vi "SDG60DeleteAllWaveforms.vi"(2 "error in (no error)":errorcluster, 4 "VISA resource name":refnum<visa-resource-name>="USB0::0xF4EC::0x1101::SDG6XEBC5R0119::INSTR") -> (0 "error out":errorcluster, 1 "VISA resource name out":refnum<visa-resource-name>, 3 "Time Estimation (s)":i32=7 format="%.15f")   [LabVIEW 2018]
doc: "Establishes communication with the instrument and optionally performs an instrument identification query and/or an instrument reset. It also places the instrument in a default state needed for other instrument driver operations. Therefore, call this VI before calling other instrument driver VIs for this instrument. Generally, you need to call the Initialize VI only once at the beginning of an application."
panel:
  out "All deleted":bool
  out "Number of Waveforms":i32=7
  out "WFM Names":string
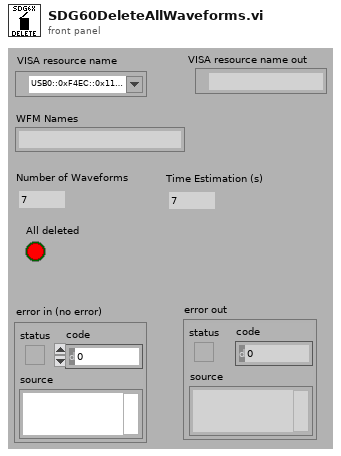
[diagram p1: front panel]
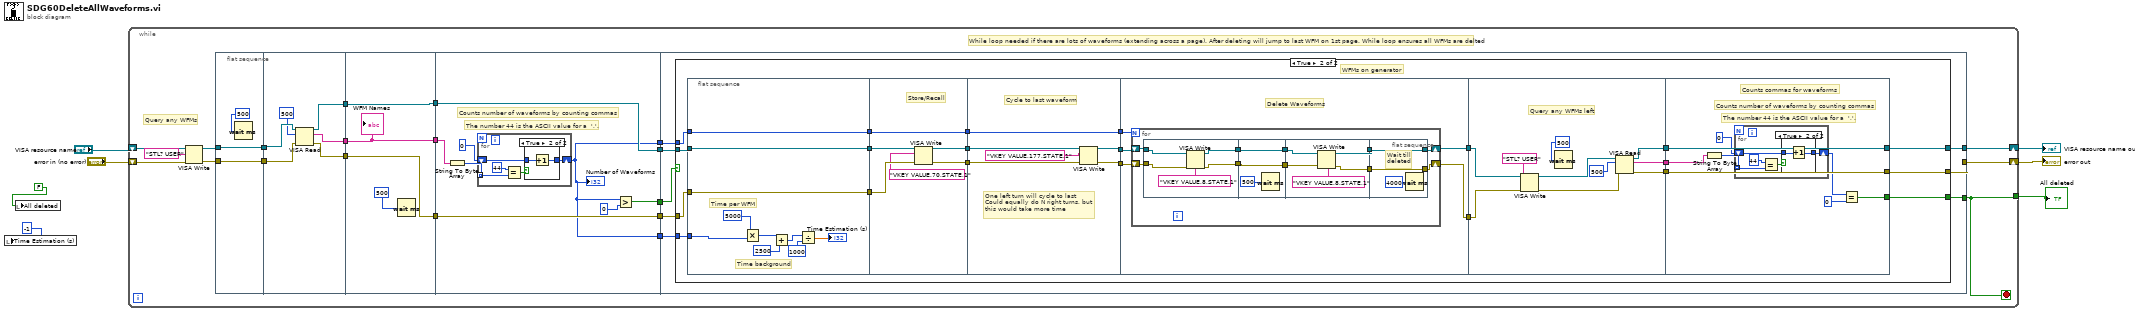
[diagram p0: block diagram]
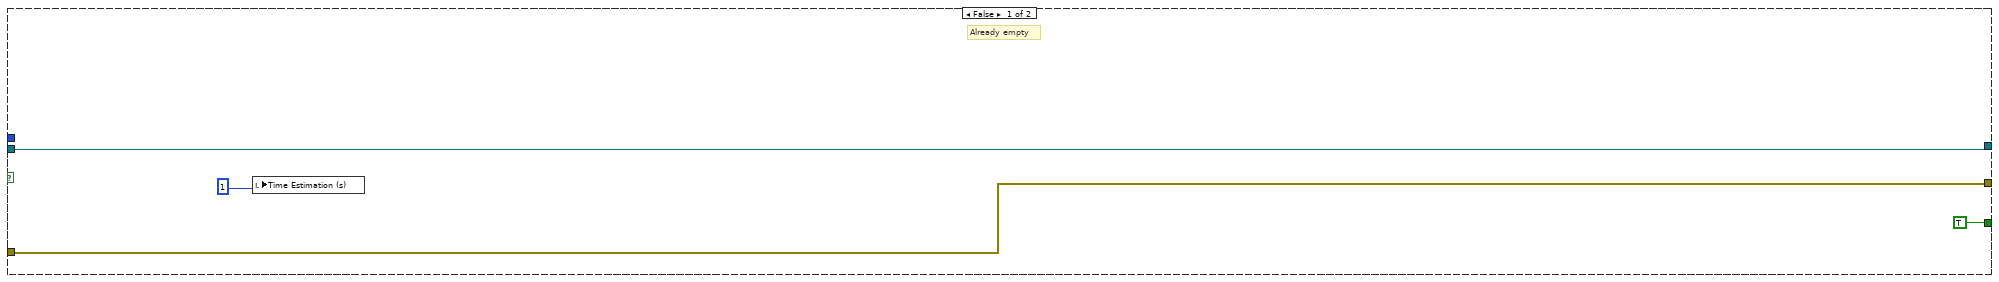
[diagram p3: hidden frame]
diagram:
  n1 = local write "Time Estimation (s)"(-1) -> ()
  n2 = local write "All deleted"(FALSE) -> ()
  n3 = while {
    shift-right: [w14] -> w4
    shift-left: "VISA resource name" -> [w11]
    shift-right: [w15] -> w5
    shift-left: "error in (no error)" -> [w13]
    tunnel: [w8] -> w1
    stop <- w8 stop-if-true
    # "While loop needed if there are lots of waveforms (extending across a page). After deleting will jump to last WFM on 1st page. While loop ensures all WFMs are delted"
    # "Query any WFMs"
    n4 = VISA Write(VISA resource name=w11, write buffer="STL? USER", error in (no error)=w13) -> (VISA resource name out=w9:refnum<visa-resource-name>, error out=w10:errorcluster)  [unwired: 1 out]
    n5 = flat-sequence {
      tunnel: [w31] -> w28
      tunnel: [w30] -> w27
      tunnel: w9 -> [w31]
      tunnel: w10 -> [w30]
      tunnel: w28 -> [w37]
      tunnel: w27 -> [w34]
      tunnel: [w36] -> w26
      tunnel: [w35] -> w25
      tunnel: [w32] -> w24
      tunnel: w26 -> [w41]
      tunnel: w25 -> [w40]
      tunnel: w24 -> [w38]
      tunnel: [w41] -> w23
      tunnel: [w40] -> w22
      tunnel: [w38] -> w21
      tunnel: w23 -> [w49]
      tunnel: w22 -> [w48]
      tunnel: w21 -> [w45]
      tunnel: [w49] -> w20
      tunnel: [w48] -> w19
      tunnel: [w44] -> w18
      tunnel: [w44] -> w17
      tunnel: [w42] -> w16
      tunnel: w20 -> [w64]
      tunnel: w19 -> [w63]
      tunnel: w18 -> [w65]
      tunnel: [w62] -> w15
      tunnel: [w61] -> w14
      tunnel: w17 -> [w60]
      tunnel: w16 -> [w59]
      tunnel: [w58] -> w8
      frame #0 {
        n6 = Wait (ms)(milliseconds to wait=500) -> ()  [unwired: 1 out]
      }
      frame #1 {
        n7 = VISA Read(VISA resource name=w37, byte count=500, error in (no error)=w34) -> (VISA resource name out=w36:refnum<visa-resource-name>, read buffer=w32:string, error out=w35:errorcluster)  [unwired: 1 out]
      }
      frame #2 {
        n8 = Wait (ms)(milliseconds to wait=500) -> ()  [unwired: 1 out]
        "WFM Names" <- w38
      }
      frame #3 {
        # "Counts number of waveforms by counting commas"
        # "The number 44 is the ASCII value for a  ','."
        n9 = String To Byte Array(string=w45) -> (unsigned byte array=w47:u8[])
        n10 = for {
          shift-right: [w52] -> w44
          shift-left: 0 -> [w53]
          tunnel: w47 -> [w51] mode=indexing
          n11 = Equal?(x=u8 44, y=w51) -> (x = y?=w54:bool)
          n12 = case shown="True" w54 {
            tunnel: w53 -> [w55 w57]
            tunnel: [w55 w56] -> w52
            frame False {
            }
            frame True {
              n13 = Increment(x=w57) -> (x+1=w56:i32)
            }
          }
        }
        "Number of Waveforms" <- w44
        n14 = Greater?(x=w44, y=0) -> (0:w42:bool)
      }
      frame #4 {
        n15 = case shown="True" w59 {
          tunnel: w65 -> [_ w76]
          tunnel: w64 -> [w69 w75]
          tunnel: w63 -> [w67 w74]
          tunnel: [w67 w73] -> w62
          tunnel: [w69 w72] -> w61
          tunnel: w60 -> [_ w71]
          tunnel: [TRUE w70] -> w58
          frame False {
            # "Already empty"
            n16 = local write "Time Estimation (s)"(1) -> ()
          }
          frame True {
            # "WFMs on generator"
            n17 = flat-sequence {
              tunnel: w74 -> [w98]
              tunnel: w75 -> [w99]
              tunnel: w76 -> [w100]
              tunnel: [w100] -> w90
              tunnel: [w99] -> w89
              tunnel: [w98] -> w88
              tunnel: w71 -> [w93]
              tunnel: [w106] -> w87
              tunnel: [w102] -> w86
              tunnel: [w101] -> w85
              tunnel: w90 -> [w106]
              tunnel: w89 -> [w105]
              tunnel: w88 -> [w104]
              tunnel: w87 -> [w112]
              tunnel: w86 -> [w110]
              tunnel: w85 -> [w111]
              tunnel: [w112] -> w84
              tunnel: [w108] -> w83
              tunnel: [w109] -> w82
              tunnel: w84 -> [w117]
              tunnel: w83 -> [w113]
              tunnel: w82 -> [w116]
              tunnel: [w115] -> w81
              tunnel: [w114] -> w80
              tunnel: w81 -> [w145]
              tunnel: w80 -> [w149]
              tunnel: [w151] -> w79
              tunnel: [w150] -> w78
              tunnel: [w144] -> w77
              tunnel: [w160] -> w72
              tunnel: [w161] -> w73
              tunnel: w79 -> [w161]
              tunnel: w78 -> [w160]
              tunnel: w77 -> [w157]
              tunnel: [w154] -> w70
              frame #0 {
                # "Time background"
                # "Time per WFM"
                n18 = Multiply(x=5000, y=w93) -> (x*y=w96:i32)
                n19 = Add(x=w96, y=2500) -> (x+y=w92:i32)
                n20 = Divide(x=w92, y=1000) -> (x/y=→"Time Estimation (s)":dbl)
              }
              frame #1 {
                # "Store/Recall"
                n21 = VISA Write(VISA resource name=w105, write buffer="VKEY VALUE,70,STATE,1", error in (no error)=w104) -> (VISA resource name out=w102:refnum<visa-resource-name>, error out=w101:errorcluster)  [unwired: 1 out]
              }
              frame #2 {
                # "One left turn will cycle to last\nCould equally do N right turns, but \nthis would take more time"
                # "Cycle to last waveform"
                n22 = VISA Write(VISA resource name=w110, write buffer="VKEY VALUE,177,STATE,1", error in (no error)=w111) -> (VISA resource name out=w108:refnum<visa-resource-name>, error out=w109:errorcluster)  [unwired: 1 out]
              }
              frame #3 {
                # "Delete Waveforms"
                n23 = for {
                  N: w117 -> [_]
                  shift-right: [w126] -> w115
                  shift-left: w113 -> [w118]
                  shift-right: [w119] -> w114
                  shift-left: w116 -> [w127]
                  n24 = flat-sequence {
                    tunnel: w127 -> [w132]
                    tunnel: w118 -> [w131]
                    tunnel: [w130] -> w125
                    tunnel: [w128] -> w122
                    tunnel: w125 -> [w135]
                    tunnel: [w135] -> w124
                    tunnel: [w133] -> w123
                    tunnel: w122 -> [w133]
                    tunnel: w124 -> [w139]
                    tunnel: w123 -> [w136]
                    tunnel: [w138] -> w121
                    tunnel: [w137] -> w120
                    tunnel: [w143] -> w126
                    tunnel: w121 -> [w143]
                    tunnel: w120 -> [w141]
                    tunnel: [w141] -> w119
                    frame #0 {
                      n25 = VISA Write(VISA resource name=w131, write buffer="VKEY VALUE,8,STATE,1", error in (no error)=w132) -> (VISA resource name out=w130:refnum<visa-resource-name>, error out=w128:errorcluster)  [unwired: 1 out]
                    }
                    frame #1 {
                      n26 = Wait (ms)(milliseconds to wait=500) -> ()  [unwired: 1 out]
                    }
                    frame #2 {
                      n27 = VISA Write(VISA resource name=w139, write buffer="VKEY VALUE,8,STATE,1", error in (no error)=w136) -> (VISA resource name out=w138:refnum<visa-resource-name>, error out=w137:errorcluster)  [unwired: 1 out]
                    }
                    frame #3 {
                      # "Wait till\ndeleted"
                      n28 = Wait (ms)(milliseconds to wait=4000) -> ()  [unwired: 1 out]
                    }
                  }
                }
              }
              frame #4 {
                # "Query any WFMs left"
                n29 = VISA Write(VISA resource name=w145, write buffer="STL? USER", error in (no error)=w149) -> (VISA resource name out=w147:refnum<visa-resource-name>, error out=w146:errorcluster)  [unwired: 1 out]
                n30 = Wait (ms)(milliseconds to wait=500) -> ()  [unwired: 1 out]
                n31 = VISA Read(VISA resource name=w147, byte count=500, error in (no error)=w146) -> (VISA resource name out=w150:refnum<visa-resource-name>, read buffer=w144:string, error out=w151:errorcluster)  [unwired: 1 out]
              }
              frame #5 {
                # "Counts commas for waveforms"
                # "Counts number of waveforms by counting commas"
                # "The number 44 is the ASCII value for a  ','."
                n32 = String To Byte Array(string=w157) -> (unsigned byte array=w159:u8[])
                n33 = for {
                  shift-right: [w164] -> w156
                  shift-left: 0 -> [w165]
                  tunnel: w159 -> [w163] mode=indexing
                  n34 = Equal?(x=u8 44, y=w163) -> (x = y?=w166:bool)
                  n35 = case shown="True" w166 {
                    tunnel: w165 -> [w167 w169]
                    tunnel: [w167 w168] -> w164
                    frame False {
                    }
                    frame True {
                      n36 = Increment(x=w169) -> (x+1=w168:i32)
                    }
                  }
                }
                n37 = Equal?(x=w156, y=0) -> (x = y?=w154:bool)
              }
            }
          }
        }
      }
    }
  }
  "VISA resource name out" <- w4
  "error out" <- w5
  "All deleted" <- w1
